vi "get_fpga_version.vi"(8 "error in":errorcluster, 9 "I2C interface":T1) -> (0 "error out":errorcluster, 3 "FPGA code version":i16)   [LabVIEW 2012]
uses:
  i2c_interface.ctl
  fpga_reference.ctl
  <vilib>/Utility/error.llb/Error Cluster From Error Code.vi
  <vilib>/rvi/errors/niLvFpgaAdjustHostInterfaceError.vi
  <vilib>/rvi/interface/nirviReadWriteControl/nirviReadWriteControl.xnode
  FPGA Bitfiles/i2cmuxdemux.lvbitx
  FPGA/i2c_mux_demux.vi
  NiFpgaLv.dll
panel:
  # "Get FPGA code version to see if we're really running the right one."
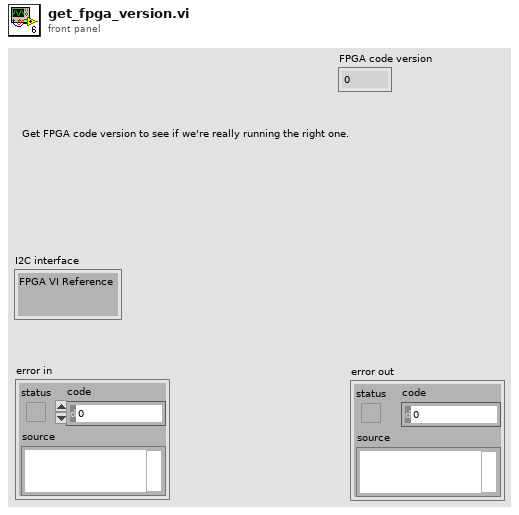
[diagram p1: front panel]
types:
  T1 = typedef "i2c_interface.ctl" = cluster{"FPGA VI Reference":T2}
  T2 = typedef "fpga_reference.ctl" = refnum<k20>
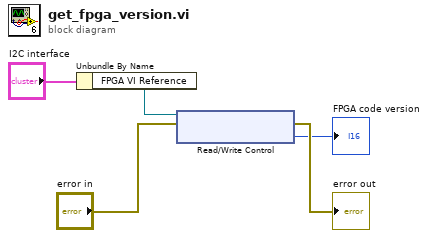
[diagram p0: block diagram]
diagram:
  n1 = Unbundle By Name("I2C interface") -> ("FPGA VI Reference"=w4:T2)
  n2 = xnode "Read/Write Control"("FPGA VI Reference In"=w4, "error in"="error in") -> ("error out"=→"error out":errorcluster, "FPGA code version"=→"FPGA code version":i16)  [unwired: 1 out]
